vi "Post_Build_Zip.vi"(8 "error in (no error)":errorcluster, 11 "Path":path) -> (0 "error out":errorcluster, 3 "Zip File":path)   [LabVIEW 2024]
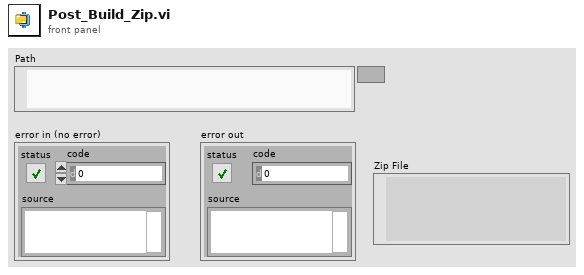
[diagram p1: front panel]
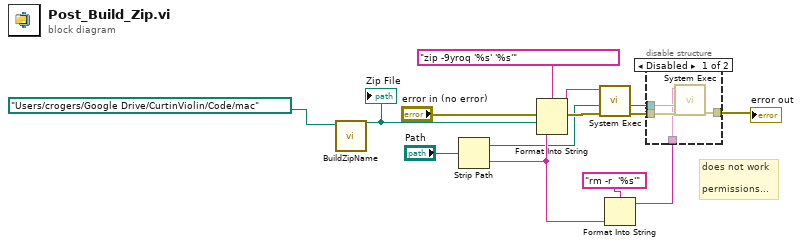
[diagram p0: block diagram]
diagram:
  # "does not work\n\npermissions..."
  n1 = call "BuildZipName.vi"("Folder"=path "/Users/crogers/Google Drive/CurtinViolin/Code/mac" ("target")) -> ("Zip File"=w1:path)  [unwired: 10 in]
  "Zip File" <- w1
  n2 = Strip Path(path="Path") -> (stripped path=w4:path, name=w5:string)
  n3 = Format Into String(format string="zip -9yroq '%s' '%s'", error in="error in (no error)", w1, w5) -> (resulting string=w9:string, error out=w10:errorcluster)  [unwired: 1 in]
  n4 = call <vilib>:"System Exec.vi"("error in (no error)"=w10, "working directory"=w4, "command line"=w9) -> ("error out"=w8:errorcluster)  [unwired: 5 in, 3 out]
  n5 = Format Into String(format string="rm -r  '%s'", w5) -> (resulting string=w3:string)  [unwired: 2 in, 1 out]
  n6 = disable-structure shown="Disabled" {
    disable-tunnel: w8 -> [w17 w18]
    disable-tunnel: [w16 w18] -> w7
    disable-tunnel: w4 -> [w15 _]
    disable-tunnel: w3 -> [w14 _]
    frame Disabled {
      n7 = call <vilib>:"System Exec.vi"("error in (no error)"=w17, "working directory"=w15, "command line"=w14) -> ("error out"=w16:errorcluster)  [unwired: 5 in, 3 out]
    }
    frame Enabled {
    }
  }
  "error out" <- w7
